vi "erode.vi"(8 "Error in":errorcluster caption="Error in (no error)", 10 "Erode Parameters (in)":T1, 11 "Erode Radio (in)":i32) -> (0 "Error out":errorcluster, 2 "Erode Parameters (out)":T1, 3 "Erode Radio (out)":i32, 4 "Erode Time (ms)":dbl)   [LabVIEW 2018]
uses:
  Controls/erode_dilate_parameters.ctl
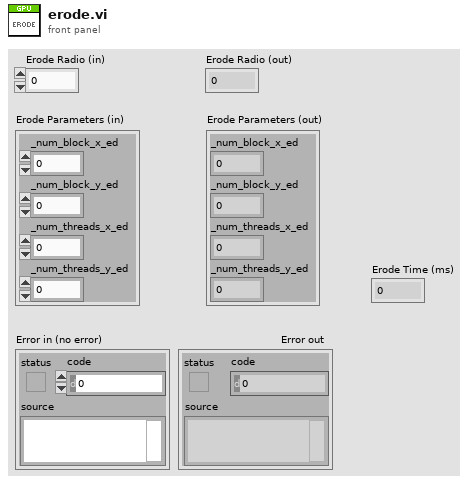
[diagram p1: front panel]
types:
  T1 = typedef "erode_dilate_parameters.ctl" = cluster{"_num_block_x_ed":i32, "_num_block_y_ed":i32, "_num_threads_x_ed":i32, "_num_threads_y_ed":i32}
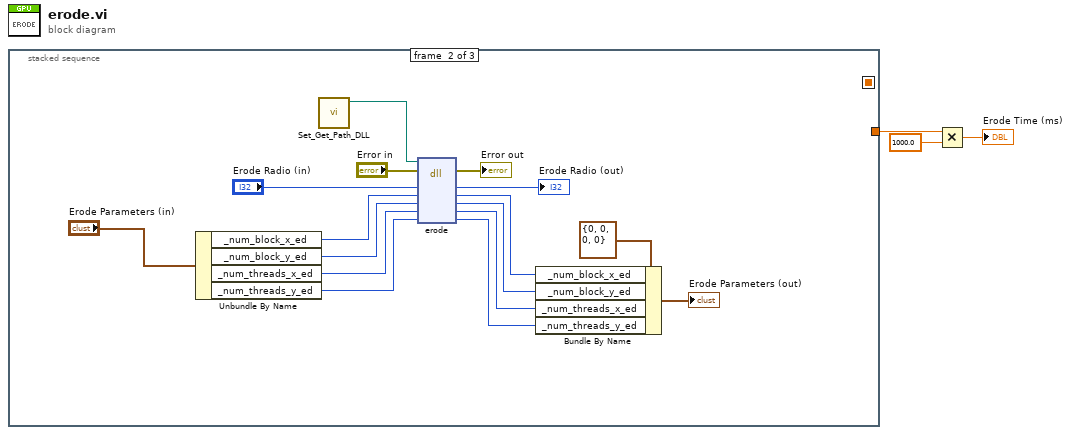
[diagram p0: block diagram]
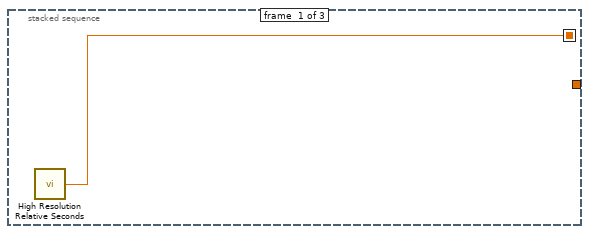
[diagram p2: hidden frame]
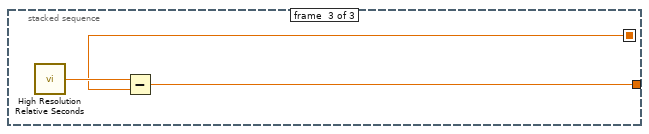
[diagram p3: hidden frame]
diagram:
  n1 = stacked-sequence {
    seq-local: [w4 _ _] -> [_ _ w22]
    tunnel: [_ _ w21] -> w1
    frame #0 {
      n2 = call <vilib>:"High Resolution Relative Seconds.vi"() -> ("relative seconds"=w4:dbl)
    }
    frame #1 {
      n3 = Unbundle By Name("Erode Parameters (in)") -> ("_num_block_x_ed"=w15:i32, "_num_block_y_ed"=w14:i32, "_num_threads_x_ed"=w13:i32, "_num_threads_y_ed"=w12:i32)
      n4 = call "Set_Get_Path_DLL.vi"() -> ("path DLL Out"=w5:path)  [unwired: 11 in]
      n5 = dll-call lib="C:/Users/AUTIS/Documents/TFG/Proyecto/Visual Studio/SR_GPU_TOOLKIT_INIT/x64/Release/SR_GPU_TOOLKIT.dll" fn="erode"(path in=w5, error in="Error in", "radio"="Erode Radio (in)", "_num_block_x_ed"=w15, "_num_block_y_ed"=w14, "_num_threads_x_ed"=w13, "_num_threads_y_ed"=w12) -> (error out=→"Error out":errorcluster, "radio"=→"Erode Radio (out)":i32, "_num_block_x_ed"=w9:i32, "_num_block_y_ed"=w8:i32, "_num_threads_x_ed"=w7:i32, "_num_threads_y_ed"=w6:i32)  [unwired: 2 in, 1 out]
      n6 = Bundle By Name(cluster=T1 {"_num_block_x_ed"=0, "_num_block_y_ed"=0, "_num_threads_x_ed"=0, "_num_threads_y_ed"=0} ("Erode & Dilate Parameters out"), "_num_block_x_ed"=w9, "_num_block_y_ed"=w8, "_num_threads_x_ed"=w7, "_num_threads_y_ed"=w6) -> (→"Erode Parameters (out)":T1)
    }
    frame #2 {
      n7 = call <vilib>:"High Resolution Relative Seconds.vi"() -> ("relative seconds"=w23:dbl)
      n8 = Subtract(x=w23, y=w22) -> (x-y=w21:dbl)
    }
  }
  n9 = Multiply(x=w1, y=1000.0) -> (x*y=→"Erode Time (ms)":dbl)
